vi "UART_Send.vi"() -> ()   [LabVIEW 2017]
uses:
  <vilib>/Instr/_visa.llb/VISA Configure Serial Port (Instr).vi
panel:
  in  "parity (0:none)":enum16{"None", "Odd", "Even", "Mark", "Space"}(ring)
  in  "data bits (8)":u16=8 min=5 max=8 step=1
  in  "flow control (0:none)":u16(ring) items=["None", "XON/XOFF", "RTS/CTS", "XON/XOFF & RTS/CTS", "DTR/DSR", "XON/XOFF & DTR/DSR"]
  in  "stop bits (10: 1 bit)":u16(ring)=10 items=["1.0"=10, "1.5"=15, "2.0"=20]
  in  "baud rate":u32=9600
  in  "milliseconds to wait":u32
  in  "stop":bool
  in  "COM port":refnum<visa-resource-name>
  out "read buffer":string
  in  "write buffer":string
  # "This app should be able to read input."
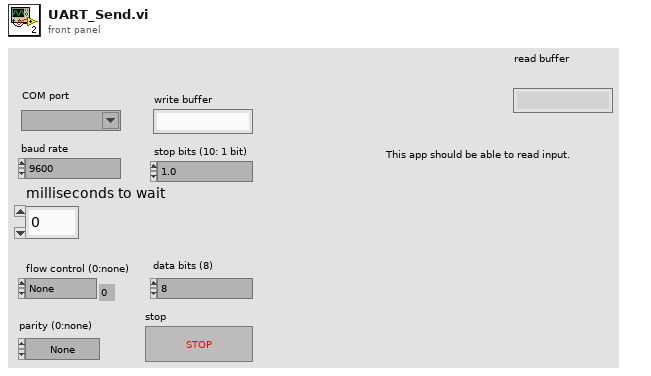
[diagram p1: front panel]
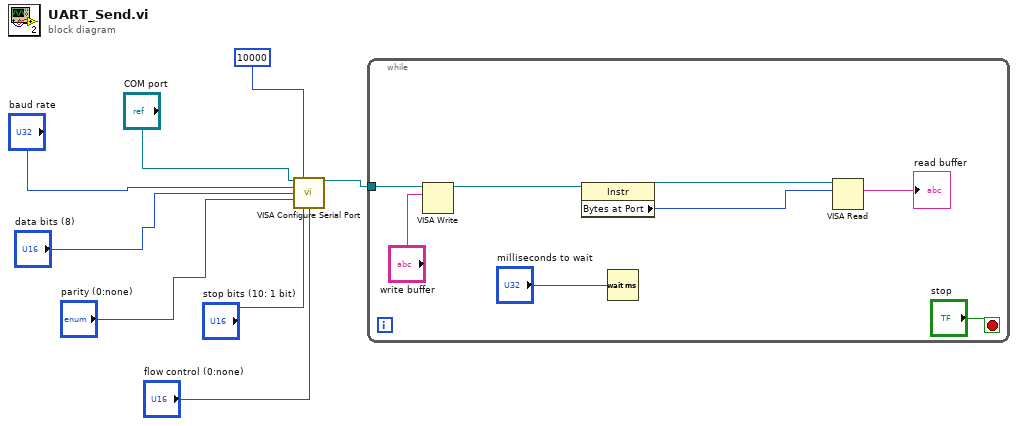
[diagram p0: block diagram]
diagram:
  n1 = call-poly "VISA Configure Serial Port"("VISA resource name"="COM port", "timeout (10sec)"=u32 10000, "baud rate (9600)"="baud rate", "data bits (8)"="data bits (8)", "parity (0:none)"="parity (0:none)", "stop bits (10: 1 bit)"="stop bits (10: 1 bit)", "flow control (0:none)"="flow control (0:none)") -> ("VISA resource name out"=w8:refnum<visa-resource-name>)  [unwired: 7 in, 1 out]
  n2 = while {
    tunnel: w8 -> [w16]
    stop <- "stop" stop-if-true
    n3 = VISA Write(VISA resource name=w16, write buffer="write buffer") -> (VISA resource name out=w15:refnum<visa-resource-name>)  [unwired: 1 in, 2 out]
    n4 = property class="Instr"(reference=w15) -> (reference out=w14:refnum<visa-resource-name>, "Bytes at Port"=w13:u32)  [unwired: 1 in, 1 out]
    n5 = Wait (ms)(milliseconds to wait="milliseconds to wait") -> ()  [unwired: 1 out]
    n6 = VISA Read(VISA resource name=w14, byte count=w13) -> (read buffer=→"read buffer":string)  [unwired: 1 in, 3 out]
  }
